vi "Read Adapters Info Registry.vi"(8 "error in (no error)":errorcluster, 10 "Array in":string[](array[string]), 11 "Numeric":i32) -> (0 "error out":errorcluster, 3 "Array":string[][](array[string]))   [LabVIEW 2015]
uses:
  <vilib>/registry/registry.llb/Registry RtKey.ctl
  <vilib>/registry/registry.llb/Registry SAM.ctl
  <vilib>/registry/registry.llb/Read Registry Value Simple STR.vi
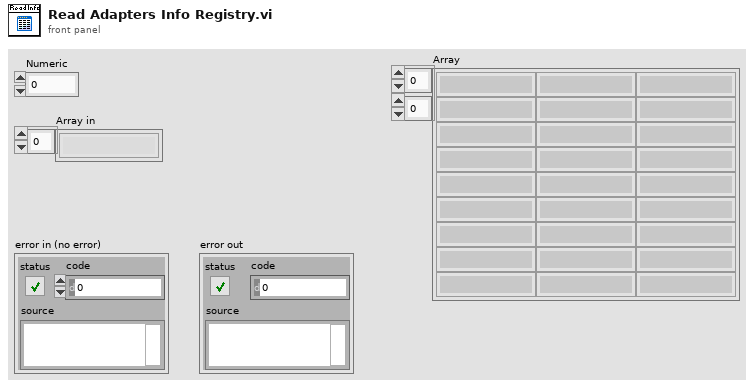
[diagram p1: front panel]
types:
  T1 = typedef "Registry SAM.ctl" = enum32{"KEY_QUERY_VALUE", "KEY_SET_VALUE", "KEY_CREATE_SUB_KEY", "KEY_ENUMERATE_SUB_KEYS", "KEY_NOTIFY", "KEY_CREATE_LINK", "KEY_READ", "KEY_WRITE", "KEY_ALL_ACCESS", "KEY_READ | KEY_WRITE"}
  T2 = typedef "Registry RtKey.ctl" = enum32{"HKEY_CLASSES_ROOT", "HKEY_CURRENT_USER", "HKEY_LOCAL_MACHINE", "HKEY_USERS", "HKEY_PERFORMANCE_DATA", "HKEY_CURRENT_CONFIG", "HKEY_DYN_DATA"}
  T3 = typedef "Registry refnum.ctl" = refnum<k1>
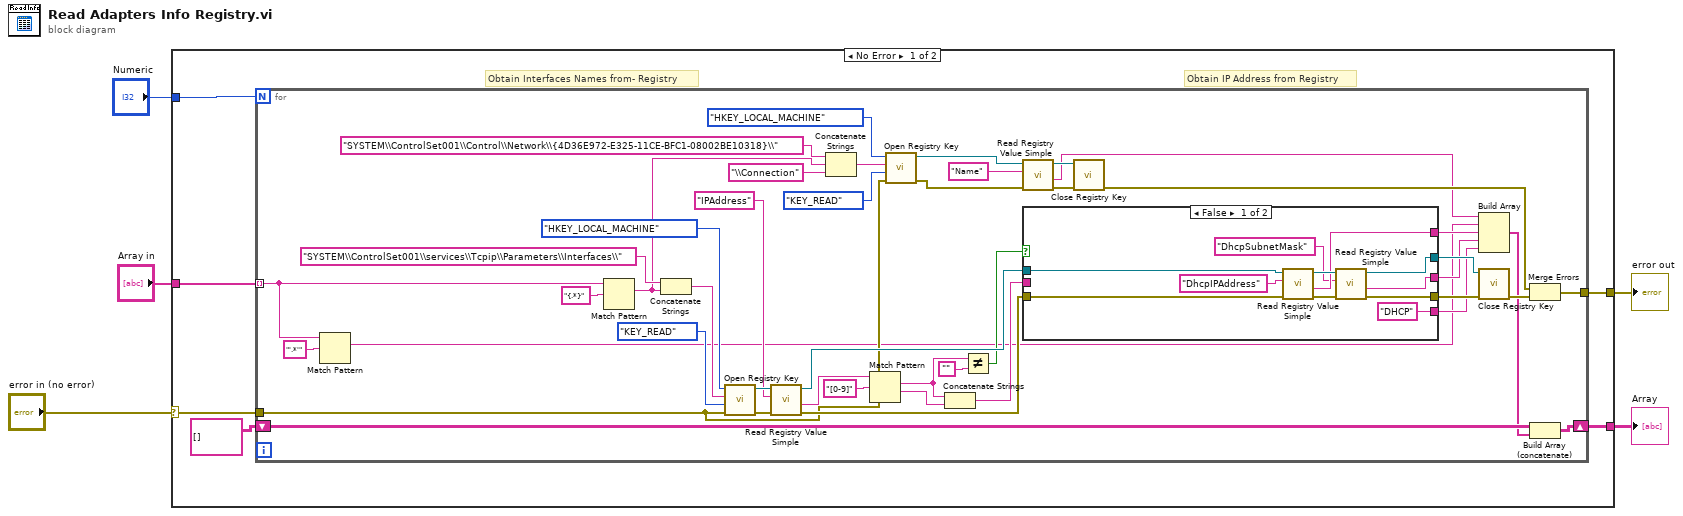
[diagram p0: block diagram]
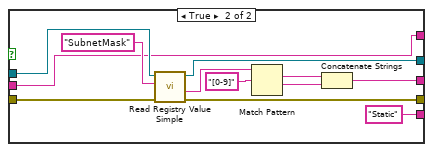
[diagram p2: hidden frame]
diagram:
  n1 = case shown="No Error" "error in (no error)" {
    selector: "error in (no error)" -> [w7 w79]
    tunnel: "Array in" -> [w11 _]
    tunnel: "Numeric" -> [w10 _]
    tunnel: [w9 _] -> w1
    tunnel: [w8 w79] -> w4
    frame No Error {
      # "Obtain IP Address from Registry"
      # "Obtain Interfaces Names from- Registry"
      n2 = for {
        N: w10 -> [_]
        tunnel: w11 -> [w43] mode=indexing
        shift-right: [w42] -> w9
        shift-left: string[][] [] -> [w41]
        tunnel: w7 -> [w20]
        tunnel: [w18] -> w8
        n3 = Match Pattern(string=w43, regular expression="'.*'") -> (match substring=w13:string)  [unwired: 1 in, 3 out]
        n4 = Match Pattern(string=w43, regular expression="{.*}") -> (match substring=w38:string)  [unwired: 1 in, 3 out]
        n5 = Concatenate Strings("SYSTEM\\ControlSet001\\services\\Tcpip\\Parameters\\Interfaces\\", w38) -> (w37:string)
        n6 = call <vilib>:"Open Registry Key.vi"("error in (no error)"=w20, "security access mask (KEY_READ | KEY_WRITE)"=Registry_SAM."KEY_READ", "subkey"=w37, "root key (HKEY_LOCAL_MACHINE)"=Registry_RtKey."HKEY_LOCAL_MACHINE") -> ("error out"=w33:errorcluster, "refnum out"=w35:T3)  [unwired: 6 in]
        n7 = call-poly <vilib>:"Read Registry Value Simple.vi"("error in (no error)"=w33, "value"="IPAddress", "refnum"=w35) -> ("error out"=w32:errorcluster, "String/Binary data"=w26:string, "refnum out"=w31:T3)  [unwired: 3 in, 1 out]
        n8 = Concatenate Strings("SYSTEM\\ControlSet001\\Control\\Network\\{4D36E972-E325-11CE-BFC1-08002BE10318}\\" ("subkey"), w38, "\\Connection" ("string")) -> (w47:string)
        n9 = Match Pattern(string=w26, regular expression="[0-9]") -> (match substring=w24:string, after substring=w23:string)  [unwired: 1 in, 2 out]
        n10 = call <vilib>:"Open Registry Key.vi"("error in (no error)"=w20, "security access mask (KEY_READ | KEY_WRITE)"=Registry_SAM."KEY_READ", "subkey"=w47, "root key (HKEY_LOCAL_MACHINE)"=Registry_RtKey."HKEY_LOCAL_MACHINE") -> ("error out"=w53:errorcluster, "refnum out"=w49:T3)  [unwired: 6 in]
        n11 = Concatenate Strings(w24, w23) -> (w22:string)
        n12 = Not Equal?(x=w24, y="") -> (x != y?=w27:bool)
        n13 = call-poly <vilib>:"Read Registry Value Simple.vi"("error in (no error)"=w53, "value"="Name", "refnum"=w49) -> ("error out"=w52:errorcluster, "String/Binary data"=w17:string, "refnum out"=w44:T3)  [unwired: 3 in, 1 out]
        n14 = case shown="False" w27 {
          tunnel: w32 -> [w63 w78]
          tunnel: w31 -> [w66 w77]
          tunnel: [w61 w75] -> w30
          tunnel: [w57 w68] -> w15
          tunnel: [w64 w74] -> w29
          tunnel: [w59 w73] -> w14
          tunnel: w22 -> [_ w73]
          tunnel: ["DHCP" "Static"] -> w16
          frame False {
            n15 = call-poly <vilib>:"Read Registry Value Simple.vi"("error in (no error)"=w63, "value"="DhcpIPAddress", "refnum"=w66) -> ("error out"=w62:errorcluster, "String/Binary data"=w59:string, "refnum out"=w65:T3)  [unwired: 3 in, 1 out]
            n16 = call-poly <vilib>:"Read Registry Value Simple.vi"("error in (no error)"=w62, "value"="DhcpSubnetMask", "refnum"=w65) -> ("error out"=w61:errorcluster, "String/Binary data"=w57:string, "refnum out"=w64:T3)  [unwired: 3 in, 1 out]
          }
          frame True {
            n17 = call-poly <vilib>:"Read Registry Value Simple.vi"("error in (no error)"=w78, "value"="SubnetMask", "refnum"=w77) -> ("error out"=w75:errorcluster, "String/Binary data"=w69:string, "refnum out"=w74:T3)  [unwired: 3 in, 1 out]
            n18 = Match Pattern(string=w69, regular expression="[0-9]") -> (match substring=w71:string, after substring=w70:string)  [unwired: 1 in, 2 out]
            n19 = Concatenate Strings(w71, w70) -> (w68:string)
          }
        }
        n20 = call <vilib>:"Close Registry Key.vi"("error in (no error)"=w52, "refnum"=w44) -> ("error out"=w21:errorcluster)  [unwired: 5 in]
        n21 = Build Array(w17, w13, w14, w15, w16) -> (w12:string[])
        n22 = call <vilib>:"Close Registry Key.vi"("error in (no error)"=w30, "refnum"=w29) -> ("error out"=w19:errorcluster)  [unwired: 5 in]
        n23 = Merge Errors(w21, w19) -> (w18:errorcluster)
        n24 = Build Array (concatenate)(w41, w12) -> (w42:string[][])
      }
    }
    frame Error {
    }
  }
  "error out" <- w4
  "Array" <- w1
